vi "CAN BOOT Get FW Info.vi"(5 "TimeOutOfMs":u32, 6 "pFWVersion":u32, 7 "pFWType":string, 9 "NAD":u8, 10 "CANIndex":i32, 11 "DevHandle":i32) -> (2 "function return":i32, 3 "pFWType out":string, 4 "pFWVersion out":u32)   [LabVIEW 2010, in "can_bootloader.lvlib"]
doc: "int WINAPI CAN_BOOT_GetFWInfo(int DevHandle,int CANIndex,unsigned char NAD,unsigned char *pFWType,unsigned int *pFWVersion,unsigned int TimeOutOfMs);"
uses:
  can_bootloader.lvlib
  USB2XXX/trunk/USB2XXX/USB2XXX/vs2010/Release/USB2XXX.dll
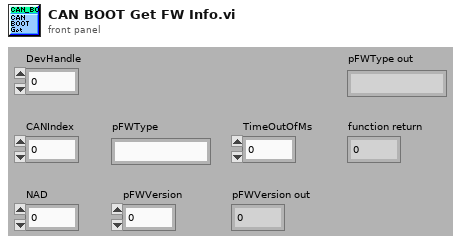
[diagram p1: front panel]
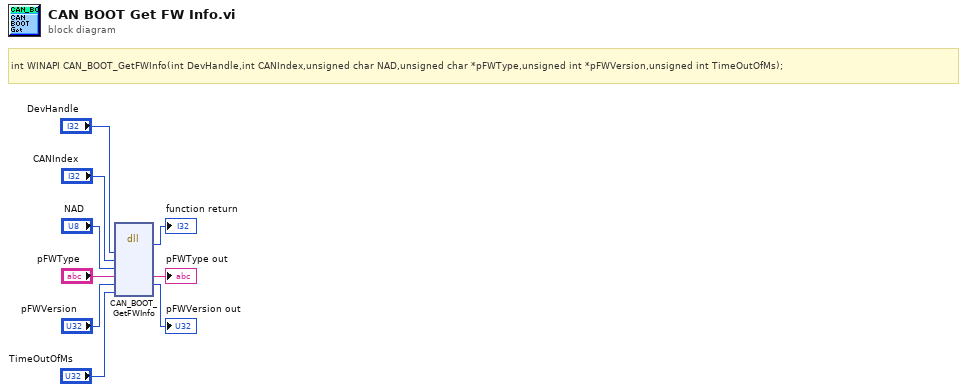
[diagram p0: block diagram]
diagram:
  # "int WINAPI CAN_BOOT_GetFWInfo(int DevHandle,int CANIndex,unsigned char NAD,unsigned char *pFWType,unsigned int *pFWVersion,unsigned int TimeOutOfMs);"
  n1 = dll-call lib="E:/OtherWork/STM32/USB2XXX/trunk/USB2XXX/USB2XXX/vs2010/Release/USB2XXX.*" fn="CAN_BOOT_GetFWInfo"("DevHandle"="DevHandle", "CANIndex"="CANIndex", "NAD"="NAD", "pFWType"="pFWType", "pFWVersion"="pFWVersion", "TimeOutOfMs"="TimeOutOfMs") -> (→"function return":i32, "pFWType"=→"pFWType out":string, "pFWVersion"=→"pFWVersion out":u32)  [unwired: 7 in, 2 out]
